vi "Test_PicoScope.vi"() -> ()   [LabVIEW 2015]
uses:
  Controls/PicoScope/pico_control_panel.ctl
  Controls/PicoScope/pico_channel_settings.ctl
  Controls/PicoScope/pico_trigger.ctl
  Controls/PicoScope/pico_init_settings.ctl
panel:
  in  "stop":bool
  in  "error in (no error)":errorcluster
  out "error out":errorcluster
  in  "PicoScope Acquisition Settings Input":T1={"Channel A Settings"={"Enabled"=TRUE, "Coupling"=1, "Range"=6, "Analogue Offset"=0.0}, "Channel B Settings"={"Enabled"=TRUE, "Coupling"=1, "Range"=6, "Analogue Offset"=0.0}, "Trigger Options"={"Trigger Enabled"=FALSE, "Trigger Source"=enum."Channel A", "Trigger Threshold (-5 to 5 V)"=0.0, "Trigger Slope"=2, "Trigger Delay (ms)"=0.0, "Auto Trigger Time (ms)"=1000}, "Pico Scope Inititalization Settings"={"USB Power"=FALSE, "Use Serial Number"=FALSE, "Resolution"=0, "Serial Number"="", "Handle"=0}, "Use PicoScope?"=FALSE, "Acquisition Settings"={"Pre Trigger Time (s)"=512.0, "Post Trigger Time (s)"=512.0, "Resolution (s)"=34.36, "Four Channel Device"=FALSE, "Number of Captures"=1.0}} {"Acquisition Settings"."Number of Captures" min=1.0 step=1.0; "Acquisition Settings"."Resolution (s)" min=8e-09 max=34.36 step=8e-09 format="%#_6p"; "Acquisition Settings"."Post Trigger Time (s)" min=0.0 format="%#_6p"; "Acquisition Settings"."Pre Trigger Time (s)" min=0.0 format="%#_6p"; "Pico Scope Inititalization Settings"."Resolution" items=["8-bit", "12-bit", "14-bit", "15-bit (max. 2 ch.)", "16-bit (max. 1 ch.)"]; "Trigger Options"."Trigger Slope" items=["Rising"=2, "Falling"=3]; "Channel B Settings"."Range" items=["10 mV", "20 mV", "50 mV", "100 mV", "200 mV", "500 mV", "1 V", "2 V", "5 V", "10 V", "20 V", "50 V ", "100 V"]; "Channel B Settings"."Coupling" items=["AC", "DC"]; "Channel A Settings"."Range" items=["10 mV", "20 mV", "50 mV", "100 mV", "200 mV", "500 mV", "1 V", "2 V", "5 V", "10 V", "20 V", "50 V ", "100 V"]; "Channel A Settings"."Coupling" items=["AC", "DC"]}
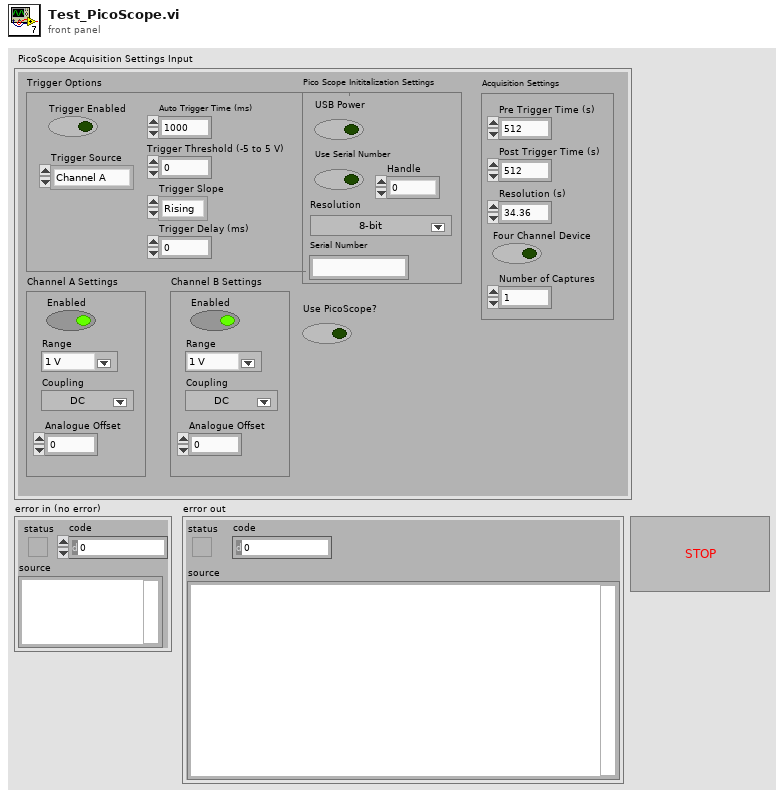
[diagram p1: front panel]
types:
  T1 = typedef "pico_control_panel.ctl" = cluster{"Channel A Settings":T2, "Channel B Settings":T2, "Trigger Options":T3, "Pico Scope Inititalization Settings":T4, "Use PicoScope?":bool, "Acquisition Settings":cluster{"Pre Trigger Time (s)":dbl, "Post Trigger Time (s)":dbl, "Resolution (s)":dbl, "Four Channel Device":bool, "Number of Captures":dbl}}
  T2 = typedef "pico_channel_settings.ctl" = cluster{"Enabled":bool, "Coupling":i16, "Range":u16, "Analogue Offset":sgl}
  T3 = typedef "pico_trigger.ctl" = cluster{"Trigger Enabled":bool, "Trigger Source":enum16{"Channel A", "Channel B", "Channel C", "Channel D", "Ext."}, "Trigger Threshold (-5 to 5 V)":dbl, "Trigger Slope":u16, "Trigger Delay (ms)":dbl, "Auto Trigger Time (ms)":i16}
  T4 = typedef "pico_init_settings.ctl" = cluster{"USB Power":bool, "Use Serial Number":bool, "Resolution":i32, "Serial Number":string, "Handle":i16}
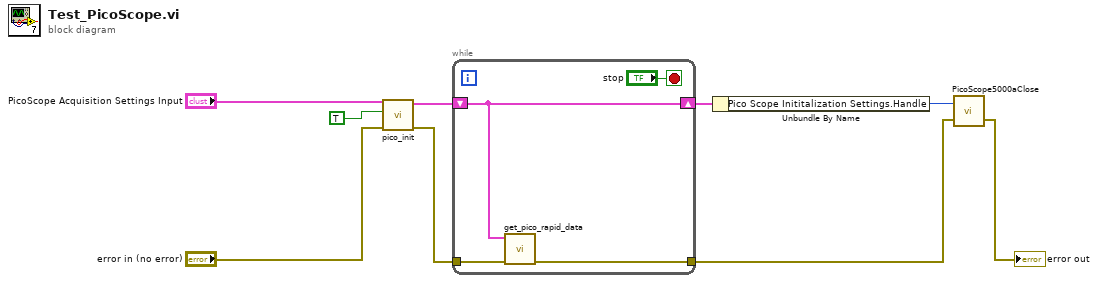
[diagram p0: block diagram]
diagram:
  n1 = call "pico_init.vi"("error in (no error)"="error in (no error)", "Initialize PicoScope?"=TRUE, "PicoScope Acquisition Settings Input"="PicoScope Acquisition Settings Input") -> ("error out"=w8:errorcluster, "PicoScope Acquisition Settings Output"=w6:T1)  [unwired: 4 in, 2 out]
  n2 = while {
    tunnel: w8 -> [w12]
    tunnel: [w11] -> w7
    shift-right: [w10] -> w3
    shift-left: w6 -> [w10]
    stop <- "stop" stop-if-true
    n3 = call "get_pico_rapid_data.vi"("error in"=w12, "PicoScope Acquisition Settings"=w10) -> ("error out"=w11:errorcluster)  [unwired: 7 in, 2 out]
  }
  n4 = Unbundle By Name(w3) -> ("Pico Scope Inititalization Settings.Handle"=w2:i16)
  n5 = call "PicoScope5000aClose.vi"("error in (no error)"=w7, "handle"=w2) -> ("error out"=→"error out":errorcluster)  [unwired: 1 in]
